vi "Convert Row of 2Chip Device.vi"(10 "cursor position":cluster{"row":i8, "column":i8}, 11 "cluster of private data in":T1={"FPGA VI Reference"=refnum, "device index"=0, "screen size"=enum."8x1", "font size"=enum."5x8", "auto wrap"=FALSE, "alignment"=enum."None", "number of line"=enum."2 lines", "shift 0"=0, "entry mode 0"=enum."increment & no shift", "shift 1"=0, "entry mode 1"=enum."increment & no shift"}) -> (1 "chip select":enum16{"1st chip", "2nd chip"}(ring), 2 "current cursor position":cluster{"row":i8, "column":i8}, 3 "cluster of private data output":T1={"FPGA VI Reference"=refnum, "device index"=0, "screen size"=enum."8x1", "font size"=enum."5x8", "auto wrap"=FALSE, "alignment"=enum."None", "number of line"=enum."2 lines", "shift 0"=0, "entry mode 0"=enum."increment & no shift", "shift 1"=0, "entry mode 1"=enum."increment & no shift"})   [LabVIEW 2017, in "HD44780.lvclass"]
uses:
  HD44780.lvclass
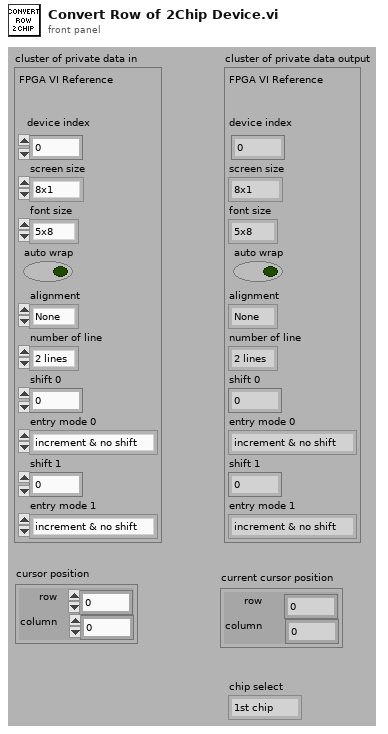
[diagram p1: front panel]
types:
  T1 = cluster{"FPGA VI Reference":refnum<k20>, "device index":i8, "screen size":enum8{"8x1", "8x2", "12x4", "16x1", "16x2", "16x4", "20x1", "20x2", "20x4", "24x1", "24x2", "40x2", "40x4"}, "font size":enum8{"5x8", "5x10"}, "auto wrap":bool, "alignment":enum16{"None", "Left", "Center", "Right"}, "number of line":enum8{"1 line", "2 lines"}, "shift 0":i8, "entry mode 0":enum8{"increment & no shift", "increment & shift", "decrement & no shift", "decrement & shift"}, "shift 1":i8, "entry mode 1":enum8{"increment & no shift", "increment & shift", "decrement & no shift", "decrement & shift"}}
  T2 = enum8{"8x1", "8x2", "12x4", "16x1", "16x2", "16x4", "20x1", "20x2", "20x4", "24x1", "24x2", "40x2", "40x4"}
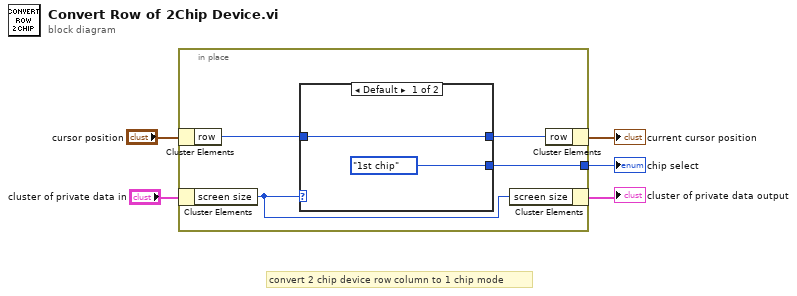
[diagram p0: block diagram]
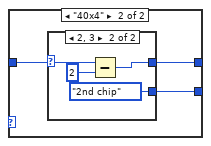
[diagram p2: hidden frame]
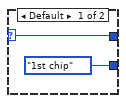
[diagram p3: hidden frame]
diagram:
  # "convert 2 chip device row column to 1 chip mode"
  n1 = in-place {
    in-place-border: [w9] -> w5
    n2 = in-place-cluster #1("cursor position") -> ("row"=w8:i8)
    n3 = in-place-cluster #2("cluster of private data in") -> ("screen size"=w6:T2)
    n4 = case shown="Default" w6 {
      tunnel: w8 -> [w10 w14]
      tunnel: [w10 w13] -> w7
      tunnel: [enum16{"1st chip", "2nd chip"}."1st chip" ("chip select  (1st chip)") w12] -> w9
      frame Default {
      }
      frame "40x4" {
        n5 = case shown="2, 3" w14 {
          selector: w14 -> [w15 w20]
          tunnel: [w15 w18] -> w13
          tunnel: [enum16{"1st chip", "2nd chip"}."1st chip" ("chip select  (1st chip)") enum16{"1st chip", "2nd chip"}."2nd chip" ("chip select  (1st chip)")] -> w12
          frame Default {
          }
          frame 2, 3 {
            n6 = Subtract(x=w20, y=i8 2) -> (x-y=w18:i8)
          }
        }
      }
    }
    n7 = in-place-cluster #2("screen size"=w6) -> (→"cluster of private data output":T1)
    n8 = in-place-cluster #1("row"=w7) -> (→"current cursor position":cluster{"row":i8, "column":i8})
  }
  "chip select" <- w5
